vi "强度图.vi"() -> ()   [LabVIEW 2012]
panel:
  out "?":i32[][](graph)
  # "距离"
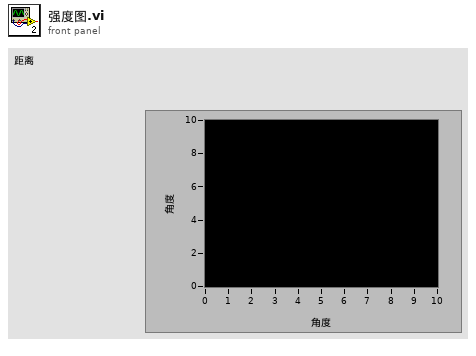
[diagram p1: front panel]
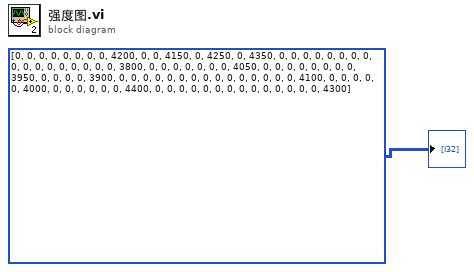
[diagram p0: block diagram]
diagram:
  "?" <- i32[][] [[0, 0, 0, 0, 0, 0, 0, 0, 4200, 0], [0, 4150, 0, 4250, 0, 4350, 0, 0, 0, 0], [0, 0, 0, 0, 0, 0, 0, 0, 0, 0], [0, 0, 0, 3800, 0, 0, 0, 0, 0, 0], [0, 4050, 0, 0, 0, 0, 0, 0, 0, 0], [3950, 0, 0, 0, 0, 3900, 0, 0, 0, 0], [0, 0, 0, 0, 0, 0, 0, 0, 0, 0], [0, 4100, 0, 0, 0, 0, 0, 4000, 0, 0], [0, 0, 0, 0, 4400, 0, 0, 0, 0, 0], [0, 0, 0, 0, 0, 0, 0, 0, 0, 4300]]
